vi "Package Builder.vi"(8 "error in":errorcluster, 10 "Build Specifications":string[](array[string]), 11 "Project Path":path) -> (0 "error out":errorcluster)   [LabVIEW 2019, in "Package Builder.lvlib"]
uses:
  Package Builder.lvlib
  TypeDefs/Post-Build Action States.ctl
  TypeDefs/Post-Build Action IDC.ctl
  <vilib>/AppBuilder/AB_API_Simple/Build (path).vi
  <vilib>/AppBuilder/AB_API_Simple/NI_App_Builder_API.lvlib
  <vilib>/National Instruments/NIPM API (Beta)/NIPM_API.lvlib
panel:
  out "Build Specification Name":string caption="String"
  out "Progress":u8(slide) scale=0.0..4.0
  out "Action":string caption="String"
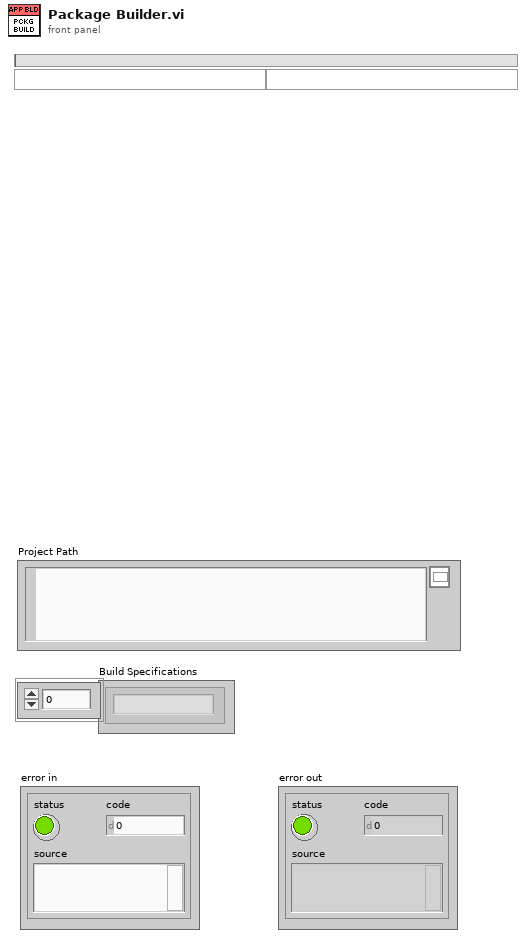
[diagram p1: front panel]
types:
  T1 = typedef "Package Builder.lvlib/Post-Build Action IDC.ctl" = cluster{"Project Path":path, "Package URL":path, "Build Specifications":string[], "Package Name":string, "Feed URL":path, "Feed Name":string, "FEEDS Folder Location":path}
  T2 = typedef "Package Builder.lvlib/Post-Build Action States.ctl" = enum16{"Initialize", "Build", "Update Feed", "Register Feed", "Open Feed", "Shutdown", "Error"}
  T3 = enum32{"Invalid", "Standard", "Closed", "Hidden", "Minimized", "Maximized"}
  T4 = enum16{"Always On", "Always Off", "Off While Running"}
  T5 = typedef "NIPM_API.lvlib/feed.ctl" = cluster{"Name":string, "URI":string}
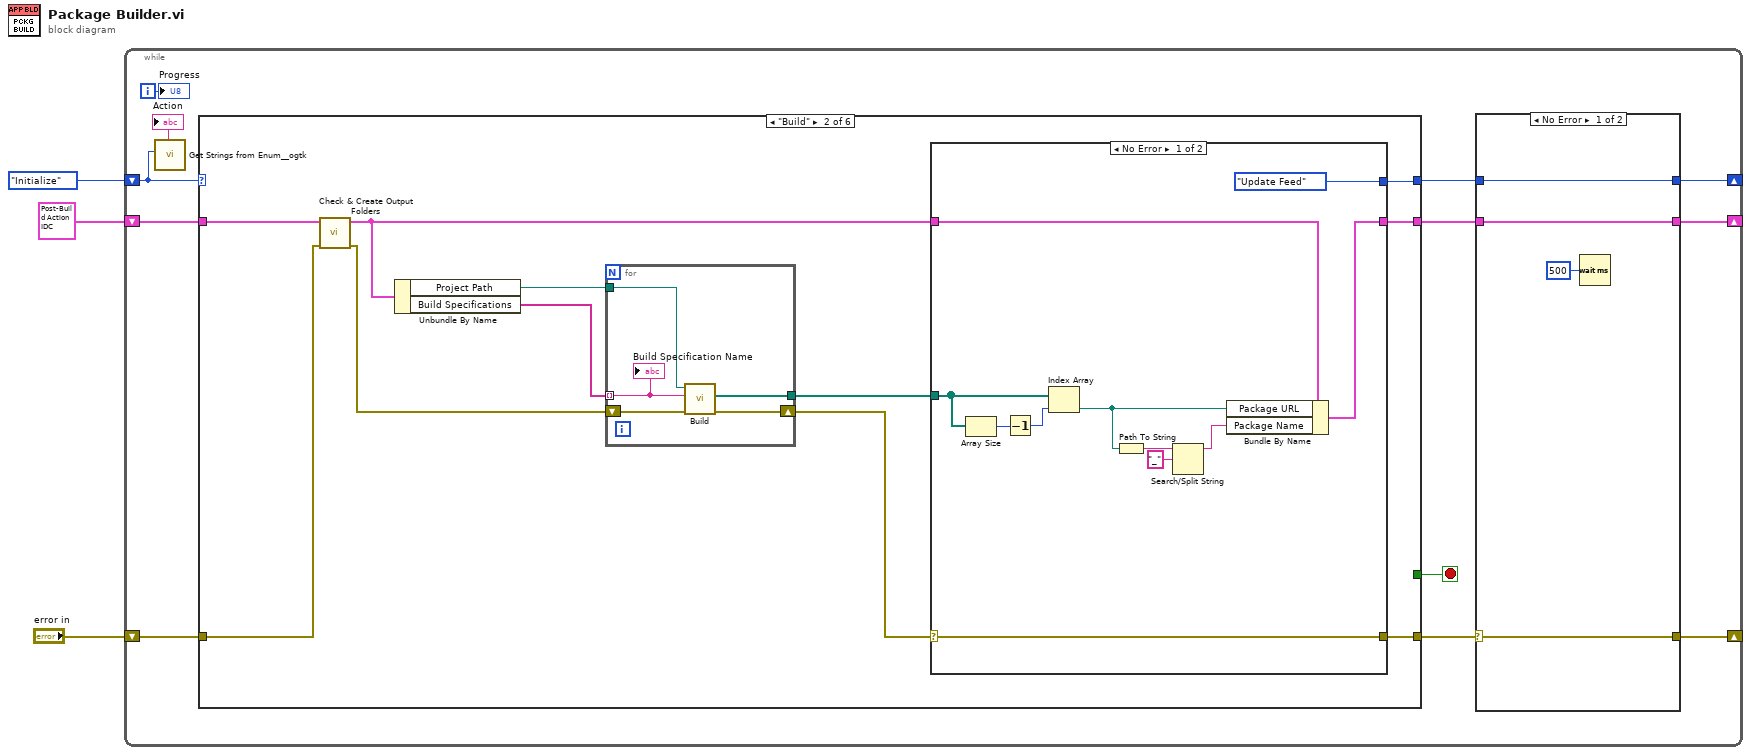
[diagram p0: block diagram]
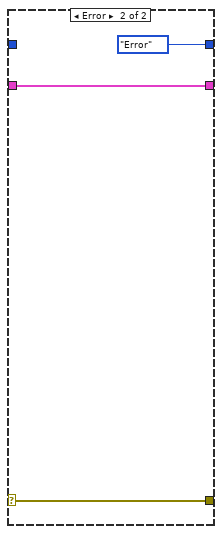
[diagram p2: hidden frame]
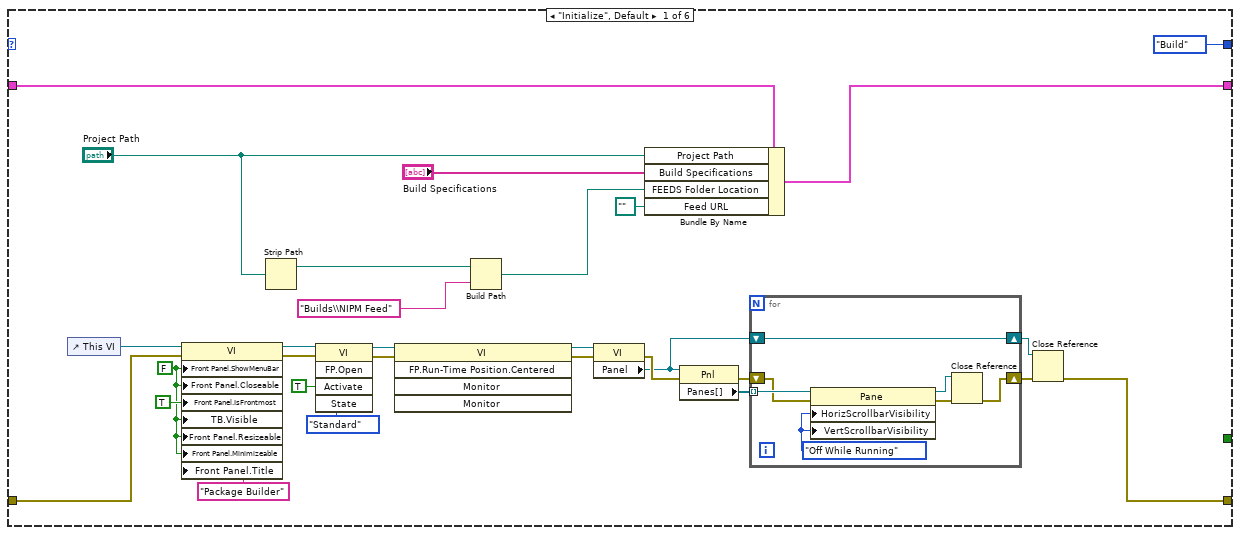
[diagram p3: hidden frame]
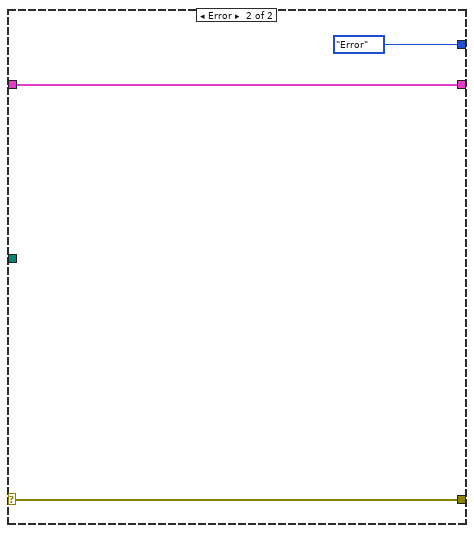
[diagram p4: hidden frame]
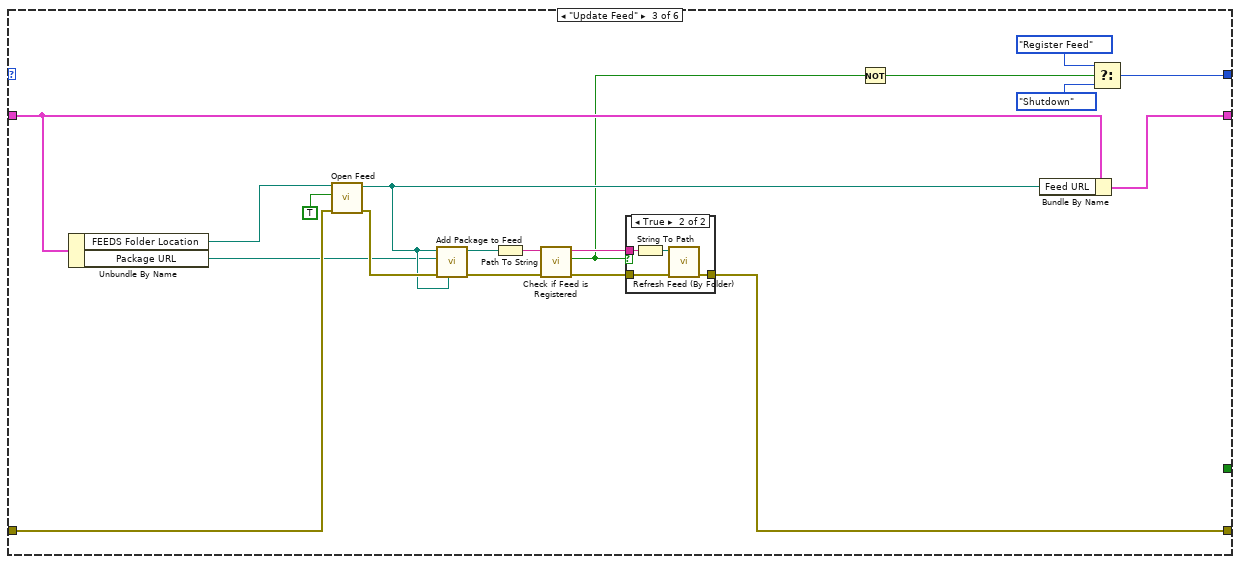
[diagram p5: hidden frame]
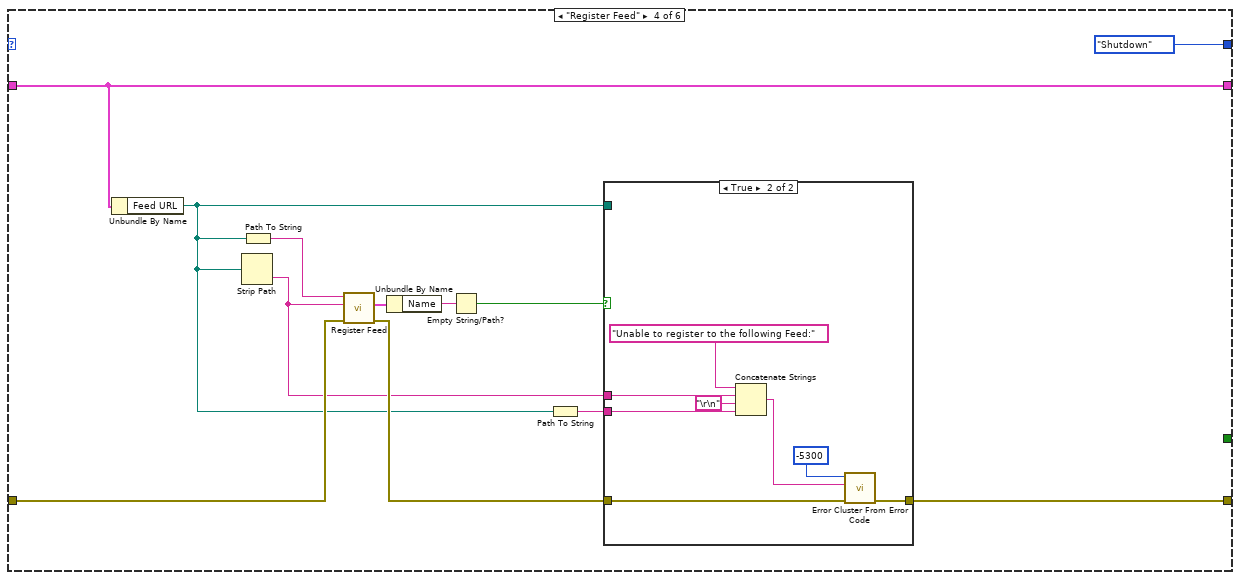
[diagram p7: hidden frame]
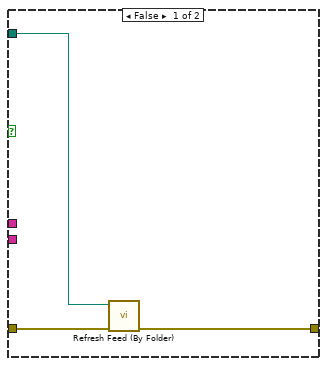
[diagram p8: hidden frame]
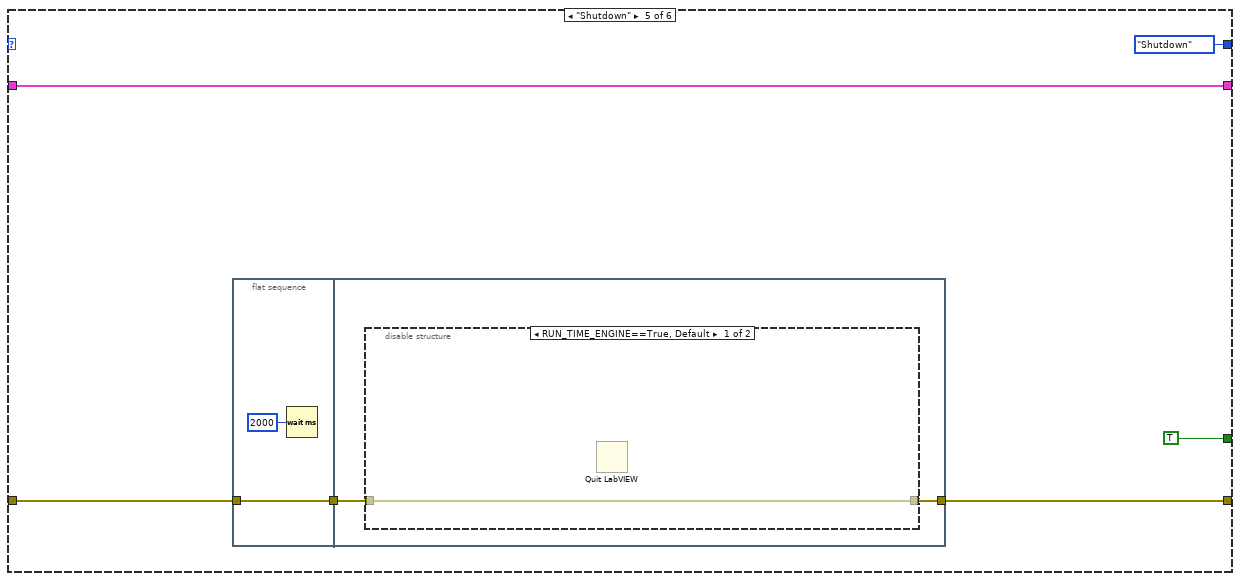
[diagram p9: hidden frame]
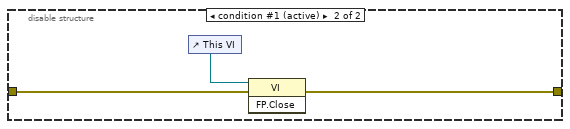
[diagram p10: hidden frame]
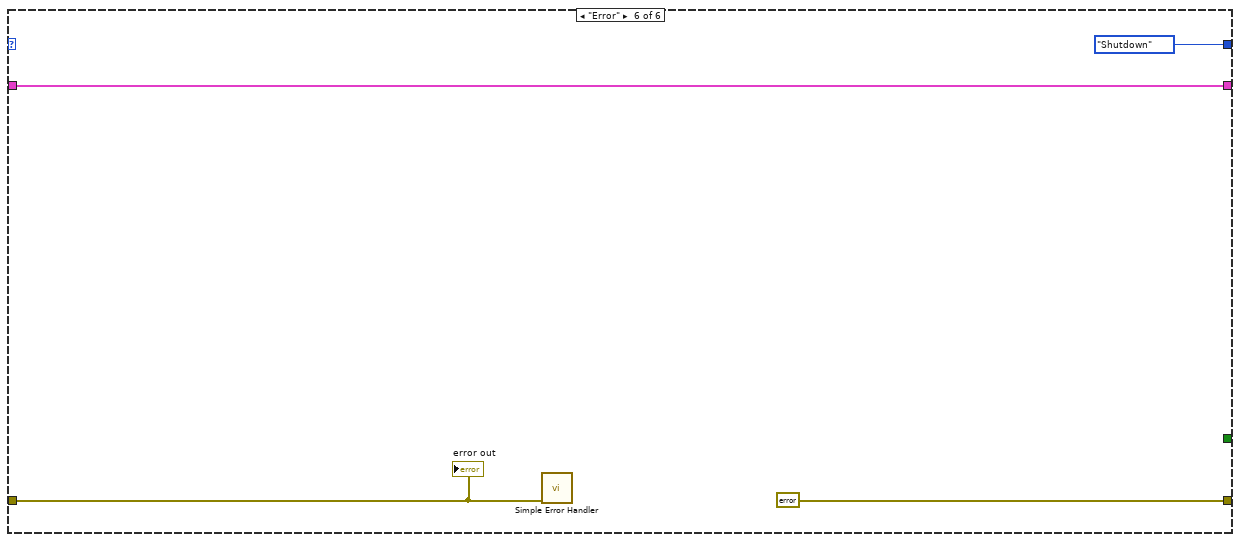
[diagram p11: hidden frame]
diagram:
  n1 = while {
    shift-right: [w14] -> _
    shift-left: Post-Build_Action_States."Initialize" -> [w5]
    shift-right: [w12] -> _
    shift-left: "error in" -> [w11]
    shift-right: [w8] -> _
    shift-left: T1 {"Project Path"=path "", "Package URL"=path "", "Build Specifications"=[], "Package Name"="", "Feed URL"=path "", "Feed Name"="", "FEEDS Folder Location"=path ""} ("Internal Data Cluster") -> [w10]
    i -> [w4]
    stop <- w7 stop-if-true
    n2 = call <userlib>:"Get Strings from Enum__ogtk.vi"("Enum"=w5) -> ("String Value"=→"Action":string)  [unwired: 7 in, 3 out]
    n3 = case shown="\"Build\"" w5 {
      tunnel: [Post-Build_Action_States."Build" w68 w98 Post-Build_Action_States."Shutdown" ("f") Post-Build_Action_States."Shutdown" ("f") Post-Build_Action_States."Shutdown" ("f")] -> w15
      tunnel: [w30 w67 w93 w116 w137 errorcluster {"status"=FALSE, "code"=0, "source"=""} ("error in")] -> w13
      tunnel: w11 -> [w31 w65 w106 w124 w138 w151]
      tunnel: w10 -> [w51 w62 w103 w123 w141 w153]
      tunnel: [w50 w69 w101 w123 w141 w153] -> w9
      tunnel: [_ _ _ _ TRUE _] -> w7
      frame "Initialize", Default {
        w33 = FALSE ("Front Panel Window:Show Menu Bar")
        n4 = control-ref of="This VI"() -> (w46:refnum<vi>)
        n5 = property class="VI"(reference=w46, error in=w31, "Front Panel.ShowMenuBar"=w33, "Front Panel.Closeable"=w33, "Front Panel.IsFrontmost"=TRUE ("Front Panel Window:Is Frontmost"), "TB.Visible"=w33, "Front Panel.Resizeable"=w33, "Front Panel.Minimizeable"=w33, "Front Panel.Title"="Package Builder" ("Front Panel Window:Title")) -> (reference out=w45:refnum<vi>, error out=w44:errorcluster)
        n6 = Strip Path(path="Project Path") -> (stripped path=w25:path)  [unwired: 1 out]
        n7 = invoke class="VI" method="FP.Open"(reference=w45, error in=w44, "Activate"=TRUE ("Activate?"), "State"=T3."Standard") -> (reference out=w47:refnum<vi>, error out=w48:errorcluster)  [unwired: 1 in, 3 out]
        n8 = invoke class="VI" method="FP.Run-Time Position.Centered"(reference=w47, error in=w48) -> (reference out=w41:refnum<vi>, error out=w39:errorcluster)  [unwired: 3 in, 3 out]
        n9 = Build Path(base path=w25, name or relative path="Builds\\NIPM Feed") -> (appended path=w28:path)
        n10 = property class="VI"(reference=w41, error in=w39) -> (error out=w38:errorcluster, "Panel"=w35:refnum<vi>)  [unwired: 1 out]
        n11 = Bundle By Name(cluster=w51, "Project Path"="Project Path", "Build Specifications"="Build Specifications", "FEEDS Folder Location"=w28, "Feed URL"=path "") -> (w50:T1)
        n12 = property class="Pnl"(reference=w35, error in=w38) -> (error out=w37:errorcluster, "Panes[]"=w40:refnum<vi>[])  [unwired: 1 out]
        n13 = for {
          tunnel: w40 -> [w58] mode=indexing
          shift-right: [w53] -> w36
          shift-left: w37 -> [w56]
          shift-right: [w52] -> w34
          shift-left: w35 -> [w52]
          w57 = T4."Off While Running" ("Horizontal Scrollbar Visibility")
          n14 = property class="Pane"(reference=w58, error in=w56, "HorizScrollbarVisibility"=w57, "VertScrollbarVisibility"=w57) -> (reference out=w54:refnum<vi>, error out=w55:errorcluster)
          n15 = Close Reference(reference=w54, error in (no error)=w55) -> (error out=w53:errorcluster)
        }
        n16 = Close Reference(reference=w34, error in (no error)=w36) -> (error out=w30:errorcluster)
      }
      frame "Build" {
        n17 = call "Check & Create Output Folders.vi"("error in (no error)"=w65, "Internal Data Cluster in"=w62) -> ("error out"=w64:errorcluster, "Internal Data Cluster out"=w61:T1)  [unwired: 8 in]
        n18 = Unbundle By Name(w61) -> ("Project Path"=w60:path, "Build Specifications"=w59:string[])
        n19 = for {
          tunnel: [w72] -> w63
          tunnel: w60 -> [w71]
          shift-right: [w74] -> w66
          shift-left: w64 -> [w73]
          tunnel: w59 -> [w70] mode=indexing
          n20 = call-poly <vilib>:"Build.vi"("error in (no error)"=w73, "Name of build specification (if empty: build all)"=w70, "Path to project"=w71) -> ("error out"=w74:errorcluster, "Generated files"=w72:path[])  [unwired: 7 in]
          "Build Specification Name" <- w70
        }
        n21 = case shown="No Error" w66 {
          selector: w66 -> [w79 w86]
          tunnel: w61 -> [w85 w88]
          tunnel: [w81 w88] -> w69
          tunnel: [Post-Build_Action_States."Update Feed" Post-Build_Action_States."Error"] -> w68
          tunnel: [w79 w86] -> w67
          tunnel: w63 -> [w77 _]
          frame No Error {
            n22 = Array Size(array=w77) -> (size(s)=w76:i32)
            n23 = Decrement(x=w76) -> (x-1=w75:i32)
            n24 = Index Array(array=w77, index=w75) -> (element=w78:path)
            n25 = Path To String(path=w78) -> (string=w84:string)
            n26 = Search/Split String(string=w84, search string/char (-)="_") -> (substring before match=w82:string)  [unwired: 1 in, 2 out]
            n27 = Bundle By Name(cluster=w85, "Package URL"=w78, "Package Name"=w82) -> (w81:T1)
          }
          frame Error {
          }
        }
      }
      frame "Update Feed" {
        n28 = Unbundle By Name(w103) -> ("FEEDS Folder Location"=w89:path, "Package URL"=w90:path)
        n29 = call <vilib>:"Open Feed.vi"("error in"=w106, "create feed if necessary (F)"=TRUE, "feed folderpath"=w89) -> ("error out"=w105:errorcluster, "feed folderpath out"=w102:path)  [unwired: 6 in, 1 out]
        n30 = call <vilib>:"Add Package to Feed.vi"("package destination folderpath"=w102, "error in"=w105, "package source filepath"=w90, "feed folderpath in"=w102) -> ("error out"=w96:errorcluster, "feed folderpath out"=w97:path)  [unwired: 5 in, 1 out]
        n31 = Path To String(path=w97) -> (string=w104:string)
        n32 = call <vilib>:"Check if Feed is Registered.vi"("error in"=w96, "feed URI"=w104) -> ("error out"=w95:errorcluster, "feed URI registered?"=w92:bool, "feed URI out"=w94:string)  [unwired: 6 in, 1 out]
        n33 = case shown="True" w92 {
          tunnel: w95 -> [w108 w112]
          tunnel: w94 -> [_ w111]
          tunnel: [w108 w109] -> w93
          frame False {
          }
          frame True {
            n34 = String To Path(string=w111) -> (path=w110:path)
            n35 = call <vilib>:"Refresh Feed (By Folder).vi"("error in"=w112, "feed folderpath in"=w110) -> ("error out"=w109:errorcluster)  [unwired: 8 in, 1 out]
          }
        }
        n36 = Not(x=w92) -> (.not. x?=w91:bool)
        n37 = Bundle By Name(cluster=w103, "Feed URL"=w102) -> (w101:T1)
        n38 = Select(t=Post-Build_Action_States."Register Feed", s=w91, f=Post-Build_Action_States."Shutdown") -> (s? t:f=w98:T2)
      }
      frame "Register Feed" {
        n39 = Unbundle By Name(w123) -> ("Feed URL"=w113:path)
        n40 = Strip Path(path=w113) -> (name=w115:string)  [unwired: 1 out]
        n41 = Path To String(path=w113) -> (string=w121:string)
        n42 = call <vilib>:"Register Feed.vi"("error in"=w124, "feed name"=w115, "feed URI"=w121) -> ("error out"=w117:errorcluster, "registered feed"=w118:T5)  [unwired: 7 in]
        n43 = Unbundle By Name(w118) -> ("Name"=w120:string)
        n44 = Empty String/Path?(string/path=w120) -> (empty?=w119:bool)
        n45 = Path To String(path=w113) -> (string=w114:string)
        n46 = case shown="True" w119 {
          tunnel: w117 -> [w127 w135]
          tunnel: [w126 w134] -> w116
          tunnel: w115 -> [_ w129]
          tunnel: w114 -> [_ w128]
          tunnel: w113 -> [w125 _]
          frame False {
            n47 = call <vilib>:"Refresh Feed (By Folder).vi"("error in"=w127, "feed folderpath in"=w125) -> ("error out"=w126:errorcluster)  [unwired: 8 in, 1 out]
          }
          frame True {
            n48 = Concatenate Strings("Unable to register to the following Feed:" ("string"), w129, "\r\n", w128) -> (w130:string)
            n49 = call <vilib>:"Error Cluster From Error Code.vi"("error in (no error)"=w135, "error message (\"\")"=w130, "error code (0)"=-5300) -> ("error out"=w134:errorcluster)  [unwired: 6 in]
          }
        }
      }
      frame "Shutdown" {
        n50 = flat-sequence {
          tunnel: w138 -> [w143]
          tunnel: [w143] -> w136
          tunnel: [w144] -> w137
          tunnel: w136 -> [w145]
          frame #0 {
            n51 = Wait (ms)(milliseconds to wait=u32 2000) -> ()  [unwired: 1 out]
          }
          frame #1 {
            n52 = disable-structure shown="RUN_TIME_ENGINE==True, Default" {
              disable-tunnel: w145 -> [w146 w149]
              disable-tunnel: [w146 w148] -> w144
              frame condition #0 {
                n53 = Quit LabVIEW() -> ()  [unwired: 1 in]
              }
              frame condition #1 (active) {
                n54 = control-ref of="This VI"() -> (w147:refnum<vi>)
                n55 = invoke class="VI" method="FP.Close"(reference=w147, error in=w149) -> (error out=w148:errorcluster)  [unwired: 1 in, 2 out]
              }
            }
          }
        }
      }
      frame "Error" {
        n56 = call <vilib>:"Simple Error Handler.vi"("error in (no error)"=w151) -> ()  [unwired: 4 in, 5 out]
        "error out" <- w151
      }
    }
    n57 = case shown="No Error" w13 {
      selector: w13 -> [w18 w22]
      tunnel: w15 -> [w19 _]
      tunnel: [w19 Post-Build_Action_States."Error"] -> w14
      tunnel: [w18 w22] -> w12
      tunnel: w9 -> [w17 w20]
      tunnel: [w17 w20] -> w8
      frame No Error {
        n58 = Wait (ms)(milliseconds to wait=u32 500) -> ()  [unwired: 1 out]
      }
      frame Error {
      }
    }
    "Progress" <- w4
  }
